vi "ref to boolean.vi"(11 "Boolean refs":refnum<vi>[](array[refnum])) -> (2 "Boolean values":bool[](array[boolean]), 3 "Boolean refs out":refnum<vi>[](array[refnum]))   [LabVIEW 2021]
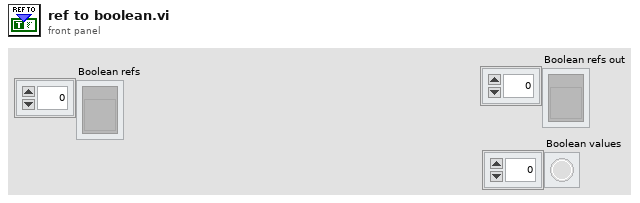
[diagram p1: front panel]
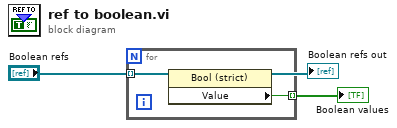
[diagram p0: block diagram]
diagram:
  n1 = for {
    tunnel: "Boolean refs" -> [w4] mode=indexing
    tunnel: [w3] -> w1 mode=indexing
    n2 = property class="Bool (strict)"(reference=w4) -> ("Value"=w3:bool)  [unwired: 1 in, 2 out]
  }
  "Boolean values" <- w1
  "Boolean refs out" <- "Boolean refs"
